vi "ErrorDefinitionSQLite_AddLibraryTest.vi"() -> ()   [LabVIEW 2018]
uses:
  ErrorDefinitionSQLite.lvclass
panel:
  in  "Size":i32
  in  "StartRange":i32
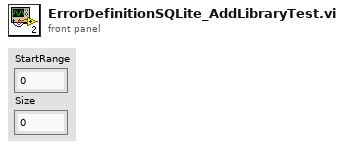
[diagram p1: front panel]
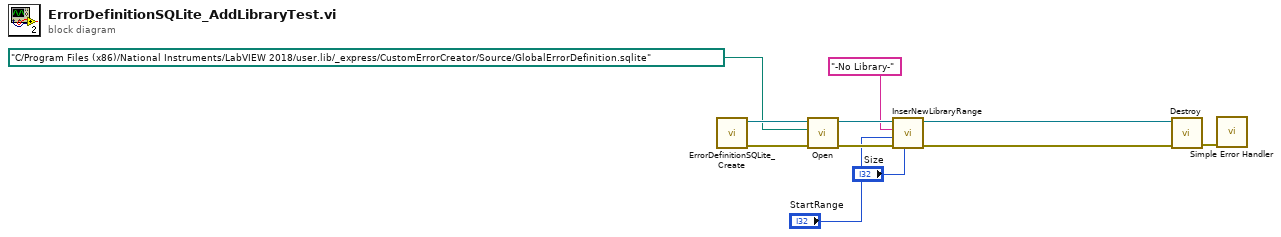
[diagram p0: block diagram]
diagram:
  n1 = call "ErrorDefinitionSQLite_Create.vi"() -> ("ErrorOut"=w10:errorcluster, "Reference out"=w11:refnum<class "ErrorDefinitionSQLite.lvclass">)  [unwired: 10 in]
  n2 = call-dynamic "Open.vi"("ErrorIn"=w10, "Path"=path "C:/Program Files (x86)/National Instruments/LabVIEW 2018/user.lib/_express/CustomErrorCreator/Source/GlobalErrorDefinition.sqlite", "ReferenceIn"=w11) -> ("ErrorOut"=w6:errorcluster, "ReferenceOut"=w7:refnum<class "ErrorDefinitionSQLite.lvclass">)  [unwired: 7 in]
  n3 = call-dynamic "InserNewLibraryRange.vi"("Size"="Size", "ErrorIn"=w6, "StartRange"="StartRange", "Library"="-No Library-", "ReferenceIn"=w7) -> ("ErrorOut"=w5:errorcluster, "ReferenceOut"=w4:refnum<class "ErrorDefinitionSQLite.lvclass">)  [unwired: 5 in]
  n4 = call-dynamic "Destroy.vi"("ErrorIn"=w5, "Reference in"=w4) -> ("ErrorOut"=w8:errorcluster)  [unwired: 8 in, 1 out]
  n5 = call <vilib>:"Simple Error Handler.vi"("error in (no error)"=w8) -> ()  [unwired: 4 in, 5 out]
